vi "InitDUTMotor.vi"(6 "CAN Signals Ref":refnum<vi>, 8 "error in (no error)":errorcluster, 9 "FetchData":T1, 10 "TPCANBaudrate":T2, 11 "DUTMotor in":refnum<class "DUTMotor.lvclass">) -> (0 "error out":errorcluster, 3 "DUTMotor out":refnum<class "DUTMotor.lvclass">)   [LabVIEW 2024, in "DUTMotor Actor.lvlib" / "DUTMotor.lvclass"]
uses:
  DUTMotor.lvclass
  ref/PCAN/CAN Communication.llb/TPCANBaudrate.ctl
  ref/PCANUSB/PCANUSB.lvclass
  DUTMotor.lvclass/DUTMotor.ctl
panel:
  in  "PCANUSB in":refnum<class "PCANUSB.lvclass">
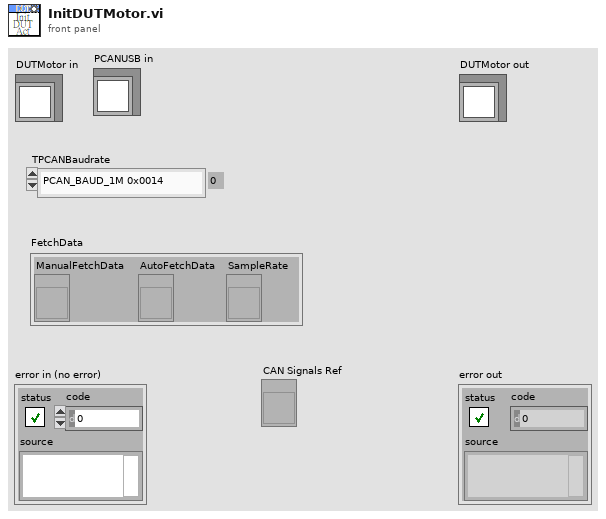
[diagram p1: front panel]
types:
  T1 = cluster{"ManualFetchData":refnum<vi>, "AutoFetchData":refnum<vi>, "SampleRate":refnum<vi>}
  T2 = typedef "TPCANBaudrate.ctl" = enum16{"PCAN_BAUD_1M 0x0014", "PCAN_BAUD_800K 0x0016", "PCAN_BAUD_500K 0x001C", "PCAN_BAUD_250K 0x011C", "PCAN_BAUD_125K 0x031C", "PCAN_BAUD_100K 0x432F", "PCAN_BAUD_95K 0xC34E", "PCAN_BAUD_83K 0x852B", "PCAN_BAUD_50K 0x472F", "PCAN_BAUD_47K 0x1414", "PCAN_BAUD_33K 0x8B2F", "PCAN_BAUD_20K 0x532F", "PCAN_BAUD_10K 0x672F", "PCAN_BAUD_5K 0x7F7F", "User Baudrate"}
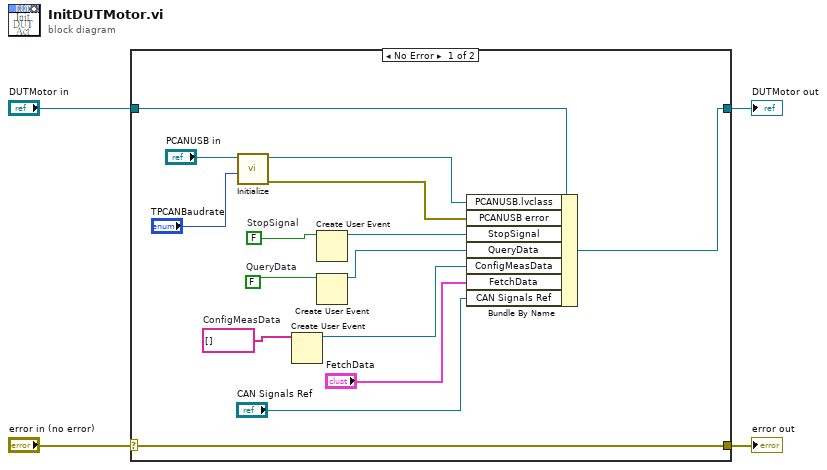
[diagram p0: block diagram]
diagram:
  n1 = case shown="No Error" "error in (no error)" {
    selector: "error in (no error)" -> [w19 w21]
    tunnel: [w19 w21] -> w3
    tunnel: [w12 w20] -> w1
    tunnel: "DUTMotor in" -> [w18 w20]
    frame No Error {
      w6 = string[] []  # ConfigMeasData
      w15 = FALSE  # QueryData
      w17 = FALSE  # StopSignal
      n2 = call "Initialize.vi"("TPCANBaudrate"="TPCANBaudrate", "PCANUSB in"="PCANUSB in") -> ("error out"=w8:errorcluster, "PCANUSB out"=w10:refnum<class "PCANUSB.lvclass">)  [unwired: 8 in]
      n3 = Create User Event(user event datatype=w6) -> (user event=w5:refnum<user-event>)  [unwired: 1 in, 1 out]
      n4 = Create User Event(user event datatype=w17) -> (user event=w16:refnum<user-event>)  [unwired: 1 in, 1 out]
      n5 = Create User Event(user event datatype=w15) -> (user event=w14:refnum<user-event>)  [unwired: 1 in, 1 out]
      n6 = Bundle By Name(cluster=w18, "PCANUSB.lvclass"=w10, "PCANUSB error"=w8, "StopSignal"=w16, "QueryData"=w14, "ConfigMeasData"=w5, "FetchData"="FetchData", "CAN Signals Ref"="CAN Signals Ref") -> (w12:refnum<class "DUTMotor.lvclass">)
    }
    frame Error {
    }
  }
  "error out" <- w3
  "DUTMotor out" <- w1
